vi "onDestroy.vi"(8 "error in (no error)":errorcluster, 11 "Pump":refnum<class "Pump.lvclass">) -> (0 "error out":errorcluster, 3 "Pump out":refnum<class "Pump.lvclass">)   [LabVIEW 2014, in "Pump.lvclass"]
doc: "JKI State Machine Objects (SMO) 1.4.0.57\nJKI - JKI\nCopyright (c) 2018, JKI"
uses:
  Pump.lvclass
  Pump.lvclass/Pump.ctl
  <vilib>/JKI/JKI SMO/SMO/SMO.lvclass
panel:
  # "For instructions on how to use the JKI State Machine Objects, examples and video tutorials, visit:\nhttp://jki.net/state-machine-objects/\n\nJKI State Machine Objects™\nhttp://jki.net/state-machine-objects/\nCopyright (C) 2005-2015, JKI <info@jki.net>\nALL RIGHTS RESERVED"
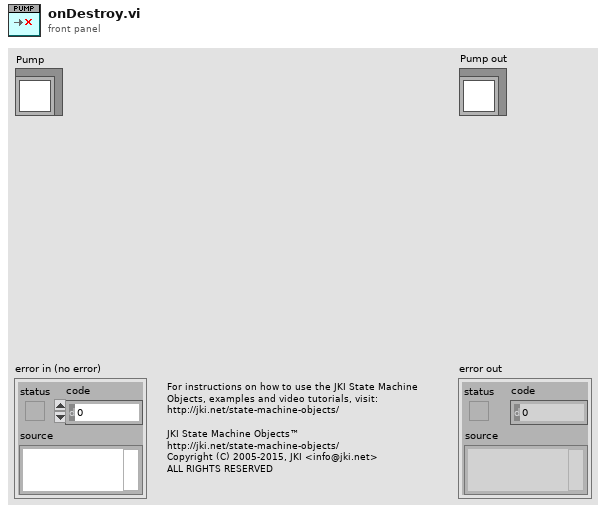
[diagram p1: front panel]
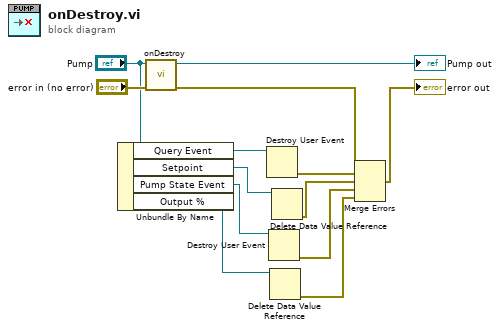
[diagram p0: block diagram]
diagram:
  n1 = Unbundle By Name("Pump") -> ("Query Event"=w10:refnum<user-event>, "Setpoint"=w5:refnum<data-value>, "Pump State Event"=w4:refnum<user-event>, "Output %"=w2:refnum<data-value>)
  n2 = call-parent "onDestroy.vi"("error in (no error)"="error in (no error)", "SMO"="Pump") -> ("error out"=w8:errorcluster, "SMO out"=→"Pump out":refnum<class "Pump.lvclass">)  [unwired: 8 in]
  n3 = Destroy User Event(user event=w10) -> (error out=w9:errorcluster)  [unwired: 1 in]
  n4 = Destroy User Event(user event=w4) -> (error out=w3:errorcluster)  [unwired: 1 in]
  n5 = Delete Data Value Reference(data value reference=w2) -> (error out=w1:errorcluster)  [unwired: 1 in, 1 out]
  n6 = Delete Data Value Reference(data value reference=w5) -> (error out=w6:errorcluster)  [unwired: 1 in, 1 out]
  n7 = Merge Errors(w8, w9, w6, w3, w1) -> (→"error out":errorcluster)
